vi "Format Coordinates.vi"(11 "1D String Array":string[](array[string])) -> (3 "Coordinates":i32[][](array[numeric]))   [LabVIEW 2019]
doc: "Given a 1D string array of points, turn them into a 2D array of coordinates."
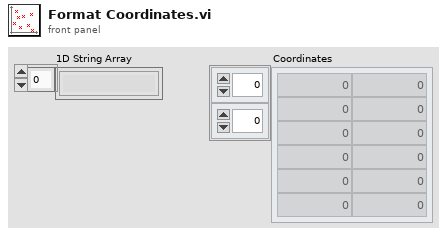
[diagram p1: front panel]
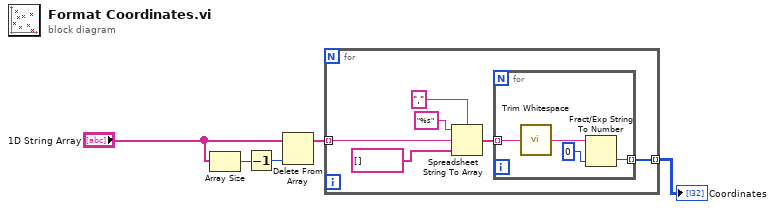
[diagram p0: block diagram]
diagram:
  n1 = Array Size(array="1D String Array") -> (size(s)=w1:i32)
  n2 = Decrement(x=w1) -> (x-1=w2:i32)
  n3 = Delete From Array(array="1D String Array", index=w2) -> (array with subset deleted=w4:string[])  [unwired: 1 in, 1 out]
  n4 = for {
    tunnel: w4 -> [w11] mode=indexing
    tunnel: [w6] -> w5 mode=indexing
    n5 = Spreadsheet String To Array(delimiter (Tab)="," ("delimiter"), format string="%s", spreadsheet string=w11, array type (2D Dbl)=string[] []) -> (array=w8:string[])
    n6 = for {
      tunnel: w8 -> [w15] mode=indexing
      tunnel: [w12] -> w6 mode=indexing
      n7 = call <vilib>:"Trim Whitespace.vi"("string"=w15) -> ("trimmed string"=w14:string)  [unwired: 1 in]
      n8 = Fract/Exp String To Number(string=w14, default (0 dbl)=0 ("default (0 DBL)")) -> (number=w12:i32)  [unwired: 2 in, 1 out]
    }
  }
  "Coordinates" <- w5
